vi "Read.vi"(8 "error in (no error)":errorcluster, 9 "Timeout (0ms)":i32, 11 "Connection Data":T1) -> (0 "error out":errorcluster, 3 "Connection Data out":T1)   [LabVIEW 2015, in "Front Panel Publisher.lvlib" / "Websocket.lvclass"]
uses:
  Websocket.lvclass
  Connection Data.ctl
  Front Panel Manager_class/Front Panel Manager.lvclass
  <vilib>/wsapi/NI_WebServices.lvlib
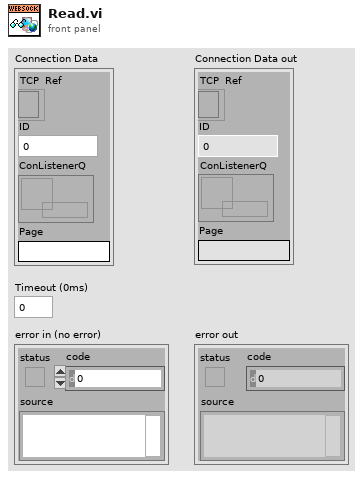
[diagram p1: front panel]
types:
  T1 = typedef "Front Panel Publisher.lvlib/Websocket.lvclass/Connection Data.ctl" = cluster{"TCP  Ref":refnum<k5>, "connection ID":u64, "ConListenerQ":refnum<queue>, "Page":string}
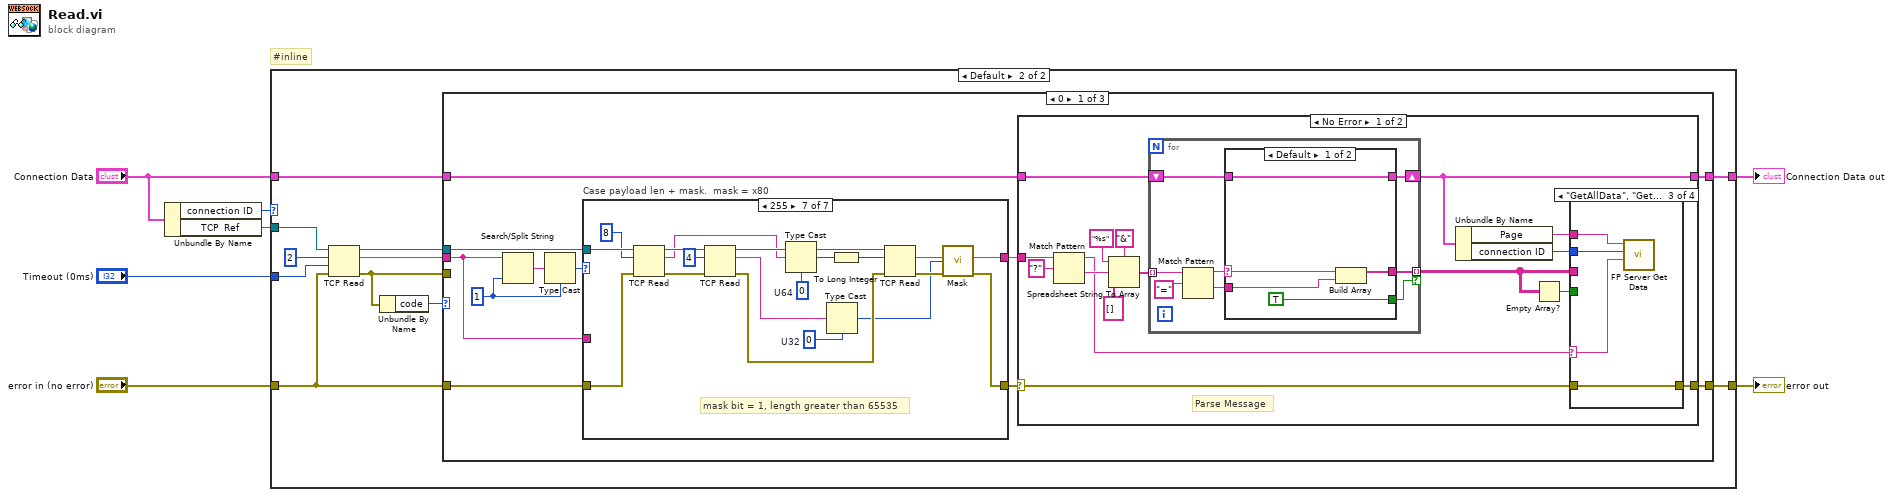
[diagram p0: block diagram]
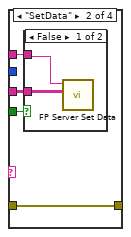
[diagram p4: hidden frame]
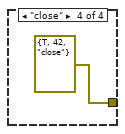
[diagram p6: hidden frame]
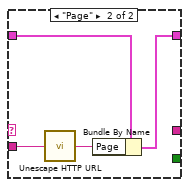
[diagram p7: hidden frame]
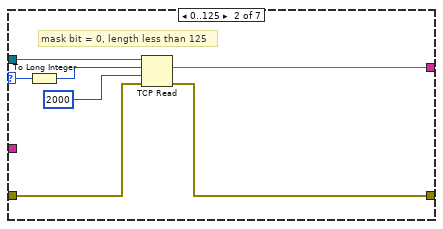
[diagram p10: hidden frame]
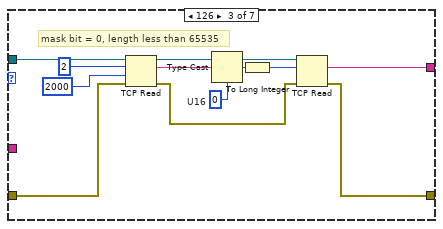
[diagram p11: hidden frame]
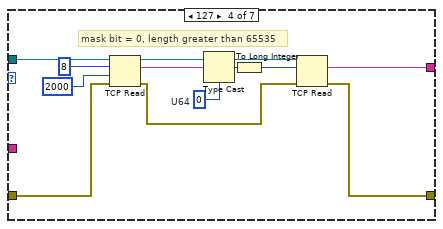
[diagram p12: hidden frame]
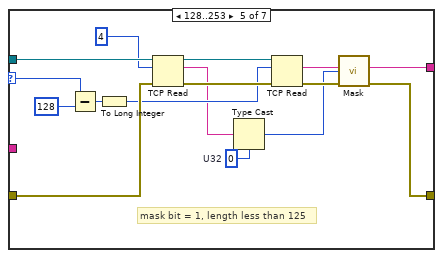
[diagram p13: hidden frame]
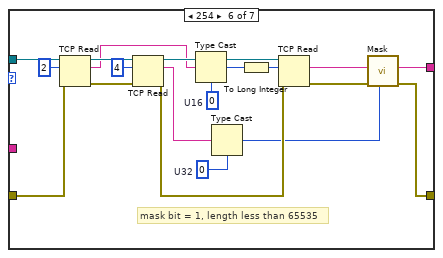
[diagram p14: hidden frame]
diagram:
  # "#inline"
  n1 = Unbundle By Name("Connection Data") -> ("connection ID"=w2:u64, "TCP  Ref"=w5:refnum<k5>)
  n2 = case shown="Default" w2 {
    tunnel: "Timeout (0ms)" -> [_ w20]
    tunnel: "error in (no error)" -> [w9 w16]
    tunnel: w5 -> [_ w15]
    tunnel: "Connection Data" -> [w8 w12]
    tunnel: [w9 w11] -> w3
    tunnel: [w8 w10] -> w1
    frame 0 {
    }
    frame Default {
      n3 = TCP Read(connection ID=w15, bytes to read=2, error in (no error)=w16, 9:w20) -> (connection ID out=w17:refnum<k5>, data out=w19:string, error out=w14:errorcluster)  [unwired: 1 in]
      n4 = Unbundle By Name(w14) -> ("code"=w13:i32)
      n5 = case shown="0" w13 {
        tunnel: w19 -> [w27 _ _]
        tunnel: w17 -> [w26 _ _]
        tunnel: [w22 w166 w168] -> w11
        tunnel: w16 -> [w31 w166 _]
        tunnel: w14 -> [_ _ w168]
        tunnel: w12 -> [w23 w165 w167]
        tunnel: [w21 w165 w167] -> w10
        frame 0 {
          w29 = u8 1 ("offset (0)")
          n6 = Search/Split String(string=w27, offset (0)=w29) -> (match + rest of string=w30:string)  [unwired: 1 in, 2 out]
          n7 = Type Cast(type=w29, x=w30) -> (*(type *) &x=w28:u8)
          n8 = case "Case payload len + mask.  mask = x80" shown="255" w28 {
            selector: w28 -> [_ w83 _ _ w121 _ _]
            tunnel: [_ w80 w87 w99 w114 w130 w149] -> w24
            tunnel: w27 -> [_ _ _ _ _ _ _]
            tunnel: w26 -> [_ w84 w95 w107 w122 w140 w159]
            tunnel: [w79 w86 w97 w109 w124 w142 w161] -> w25
            tunnel: w31 -> [w79 w85 w96 w108 w123 w141 w160]
            frame Default {
              # "error"
            }
            frame 0..125 {
              # "mask bit = 0, length less than 125"
              n9 = To Long Integer(number=w83) -> (32bit integer=w81:i32)
              n10 = TCP Read(connection ID=w84, bytes to read=w81, error in (no error)=w85, 9:2000 ("timeout ms (25000)")) -> (data out=w80:string, error out=w86:errorcluster)  [unwired: 1 in, 1 out]
            }
            frame 126 {
              w89 = u16 0  # U16
              # "mask bit = 0, length less than 65535"
              n11 = TCP Read(connection ID=w95, bytes to read=2, error in (no error)=w96, 9:2000 ("timeout ms (25000)")) -> (connection ID out=w92:refnum<k5>, data out=w91:string, error out=w98:errorcluster)  [unwired: 1 in]
              n12 = Type Cast(type=w89, x=w91) -> (*(type *) &x=w90:u16)
              n13 = To Long Integer(number=w90) -> (32bit integer=w88:i32)
              n14 = TCP Read(connection ID=w92, bytes to read=w88, error in (no error)=w98) -> (data out=w87:string, error out=w97:errorcluster)  [unwired: 2 in, 1 out]
            }
            frame 127 {
              w101 = u64 0  # U64
              # "mask bit = 0, length greater than 65535"
              n15 = TCP Read(connection ID=w107, bytes to read=8, error in (no error)=w108, 9:2000 ("timeout ms (25000)")) -> (connection ID out=w104:refnum<k5>, data out=w103:string, error out=w110:errorcluster)  [unwired: 1 in]
              n16 = Type Cast(type=w101, x=w103) -> (*(type *) &x=w102:u64)
              n17 = To Long Integer(number=w102) -> (32bit integer=w100:i32)
              n18 = TCP Read(connection ID=w104, bytes to read=w100, error in (no error)=w110) -> (data out=w99:string, error out=w109:errorcluster)  [unwired: 2 in, 1 out]
            }
            frame 128..253 {
              w112 = u32 0  # U32
              # "mask bit = 1, length less than 125"
              n19 = Subtract(x=w121, y=u8 128) -> (x-y=w117:u8)
              n20 = To Long Integer(number=w117) -> (32bit integer=w116:i32)
              n21 = TCP Read(connection ID=w122, bytes to read=4, error in (no error)=w123) -> (connection ID out=w118:refnum<k5>, data out=w113:string, error out=w126:errorcluster)  [unwired: 2 in]
              n22 = Type Cast(type=w112, x=w113) -> (*(type *) &x=w111:u32)
              n23 = TCP Read(connection ID=w118, bytes to read=w116, error in (no error)=w126) -> (data out=w115:string, error out=w125:errorcluster)  [unwired: 2 in, 1 out]
              n24 = call "Mask.vi"("mask key"=w111, "error in (no error)"=w125, "mask/unmask string in"=w115) -> ("error out"=w124:errorcluster, "mask/unmask string out"=w114:string)  [unwired: 5 in]
            }
            frame 254 {
              w128 = u32 0  # U32
              w135 = u16 0  # U16
              # "mask bit = 1, length less than 65535"
              n25 = TCP Read(connection ID=w140, bytes to read=2, error in (no error)=w141) -> (connection ID out=w138:refnum<k5>, data out=w132:string, error out=w145:errorcluster)  [unwired: 2 in]
              n26 = TCP Read(connection ID=w138, bytes to read=4, error in (no error)=w145) -> (connection ID out=w134:refnum<k5>, data out=w129:string, error out=w144:errorcluster)  [unwired: 2 in]
              n27 = Type Cast(type=w135, x=w132) -> (*(type *) &x=w136:u16)
              n28 = Type Cast(type=w128, x=w129) -> (*(type *) &x=w127:u32)
              n29 = To Long Integer(number=w136) -> (32bit integer=w133:i32)
              n30 = TCP Read(connection ID=w134, bytes to read=w133, error in (no error)=w144) -> (data out=w131:string, error out=w143:errorcluster)  [unwired: 2 in, 1 out]
              n31 = call "Mask.vi"("mask key"=w127, "error in (no error)"=w143, "mask/unmask string in"=w131) -> ("error out"=w142:errorcluster, "mask/unmask string out"=w130:string)  [unwired: 5 in]
            }
            frame 255 {
              w147 = u32 0  # U32
              w154 = u64 0  # U64
              # "mask bit = 1, length greater than 65535"
              n32 = TCP Read(connection ID=w159, bytes to read=8, error in (no error)=w160) -> (connection ID out=w157:refnum<k5>, data out=w151:string, error out=w164:errorcluster)  [unwired: 2 in]
              n33 = TCP Read(connection ID=w157, bytes to read=4, error in (no error)=w164) -> (connection ID out=w153:refnum<k5>, data out=w148:string, error out=w163:errorcluster)  [unwired: 2 in]
              n34 = Type Cast(type=w154, x=w151) -> (*(type *) &x=w155:u64)
              n35 = Type Cast(type=w147, x=w148) -> (*(type *) &x=w146:u32)
              n36 = To Long Integer(number=w155) -> (32bit integer=w152:i32)
              n37 = TCP Read(connection ID=w153, bytes to read=w152, error in (no error)=w163) -> (data out=w150:string, error out=w162:errorcluster)  [unwired: 2 in, 1 out]
              n38 = call "Mask.vi"("mask key"=w146, "error in (no error)"=w162, "mask/unmask string in"=w150) -> ("error out"=w161:errorcluster, "mask/unmask string out"=w149:string)  [unwired: 5 in]
            }
          }
          n39 = case shown="No Error" w25 {
            selector: w25 -> [w33 w78]
            tunnel: [w34 w78] -> w22
            tunnel: w24 -> [w38 _]
            tunnel: w23 -> [w47 w77]
            tunnel: [w32 w77] -> w21
            frame No Error {
              # "Parse Message"
              n40 = Match Pattern(string=w38, regular expression="?") -> (before substring=w36:string, after substring=w37:string)  [unwired: 1 in, 2 out]
              n41 = Spreadsheet String To Array(delimiter (Tab)="&", format string="%s", spreadsheet string=w37, array type (2D Dbl)=string[] []) -> (array=w42:string[])
              n42 = for {
                shift-right: [w64] -> w32
                shift-left: w47 -> [w65]
                tunnel: w42 -> [w62] mode=indexing
                tunnel: [w61] -> w41 mode=indexing if=w60
                n43 = Match Pattern(string=w62, regular expression="=") -> (before substring=w66:string, after substring=w63:string)  [unwired: 1 in, 2 out]
                n44 = case shown="Default" w66 {
                  selector: w66 -> [w70 _]
                  tunnel: w65 -> [w72 w76]
                  tunnel: [w72 w75] -> w64
                  tunnel: w63 -> [w69 w74]
                  tunnel: [TRUE _] -> w60
                  tunnel: [w68 _] -> w61
                  frame Default {
                    n45 = Build Array(w70, w69) -> (w68:string[])
                  }
                  frame "Page" {
                    n46 = call <vilib>:"Unescape HTTP URL.vi"("escaped string in"=w74) -> ("unescaped string out"=w73:string)
                    n47 = Bundle By Name(cluster=w76, "Page"=w73) -> (w75:T1)
                  }
                }
              }
              n48 = Unbundle By Name(w32) -> ("Page"=w40:string, "connection ID"=w35:u64)
              n49 = Empty Array?(array=w41) -> (empty?=w46:bool)
              n50 = case shown="\"GetAllData\", \"GetData\"" w36 {
                selector: w36 -> [_ _ w55 _]
                tunnel: w46 -> [_ w52 _ _]
                tunnel: w41 -> [_ w51 _ _]
                tunnel: w40 -> [_ w50 w58 _]
                tunnel: w35 -> [_ _ w57 _]
                tunnel: [w48 w49 w56 errorcluster {"status"=TRUE, "code"=42, "source"="close"} ("error IO")] -> w34
                tunnel: w33 -> [w48 w49 w56 _]
                frame Default {
                }
                frame "SetData" {
                  n51 = case shown="False" w52 {
                    tunnel: w51 -> [w53 _]
                    tunnel: w50 -> [w54 _]
                    frame False {
                      n52 = call "FP Server Set Data.vi"("Data"=w53, "Page"=w54) -> ()  [unwired: 9 in, 1 out]
                    }
                    frame True {
                    }
                  }
                }
                frame "GetAllData", "GetData" {
                  n53 = call "FP Server Get Data.vi"("Message"=w55, "Connection ID"=w57, "Page"=w58) -> ()  [unwired: 8 in, 1 out]
                }
                frame "close" {
                }
              }
            }
            frame Error {
            }
          }
        }
        frame 56 {
        }
        frame Default {
        }
      }
    }
  }
  "error out" <- w3
  "Connection Data out" <- w1
